vi "LABVIEW_Project.vi"() -> ()   [LabVIEW 2025]
uses:
  <vilib>/userDefined/High Color/IMAQdx.ctl
  <vilib>/MakerHub/LINX/Public/Peripherals/Analog/Analog Read 1 Chan.vi
  <vilib>/MakerHub/LINX/Public/Peripherals/Digital/Digital Write 1 Chan.vi
  <vilib>/MakerHub/LINX/Public/Peripherals/Analog/Analog Read N Chans.vi
  <vilib>/MakerHub/LINX/Public/Peripherals/Digital/Digital Write N Chans.vi
  <vilib>/MakerHub/LINX/Private/Local IO/LinxAnalogRead.vi
  <vilib>/MakerHub/LINX/Public/Utilities/Check Channel.vi
  <vilib>/MakerHub/LINX/Private/Local IO/LinxDigitalWrite.vi
  <vilib>/MakerHub/LINX/Public/Utilities/Open Serial.vi
  <vilib>/MakerHub/LINX/Private/Utilties/Generate Error.vi
  <vilib>/MakerHub/LINX/LMH-LINX.lvlib
  <vilib>/vision/driver/NI_Vision_Acquisition_Software.lvlib
panel:
  out "text":string
  in  "y":dbl=2.0 format="%#_13g"
  in  "string":string
  out "Image 2":T1(plugin-control)
  out "error out":errorcluster
  in  "Session In":T2
  out "Voltage":dbl
  out "x >= y?":bool
  in  "Serial Port":refnum<visa-resource-name>="N/A"
  in  "stop":bool
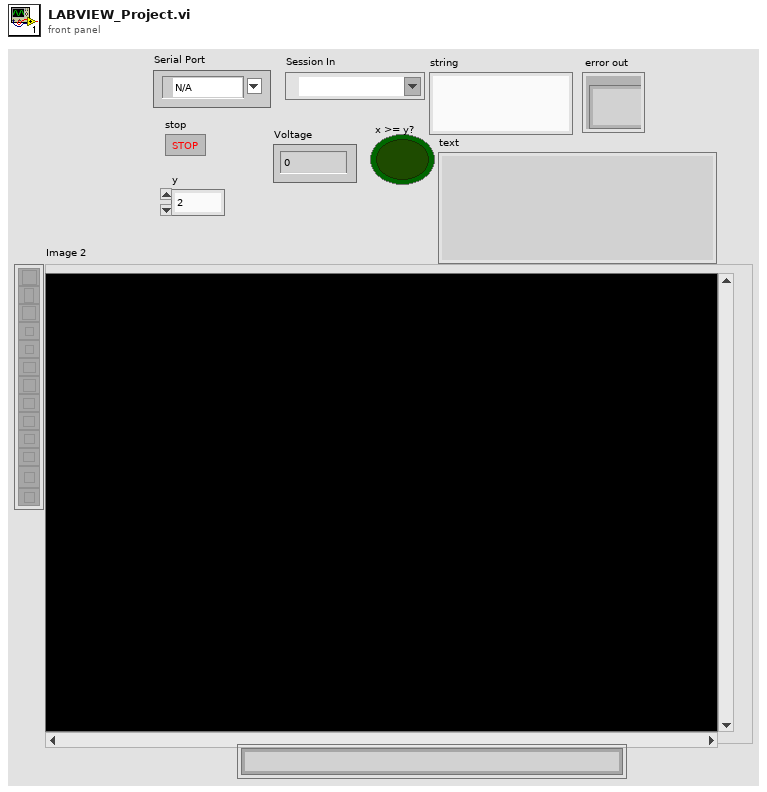
[diagram p1: front panel]
types:
  T1 = typedef "IMAQ Image.ctl" = refnum<image>
  T2 = typedef "IMAQdx.ctl" = refnum<k21>
  T3 = typedef "LMH-LINX.lvlib/LINX Ref.ctl" = cluster{"IO":T4, "Interface":T5, "LINX Device Config":T6}
  T4 = typedef "LMH-LINX.lvlib/Platform.ctl" = enum16{"Remote", "Local"}
  T5 = typedef "LMH-LINX.lvlib/Interface.ctl" = enum16{"Serial", "TCP"}
  T6 = typedef "LMH-LINX.lvlib/Device.lvlib/LINX Device Config.ctl" = cluster{"Interface":T5, "COM Port":refnum<visa-resource-name>, "TCP Configuration":T7, "Device Family":u8, "Device ID":u8, "Device Name":string, "TCP Ref":refnum<k5>, "Channels":T8}
  T7 = typedef "LMH-LINX.lvlib/Device.lvlib/TCP Config.ctl" = cluster{"IP Address":string, "Port":u16}
  T8 = typedef "LMH-LINX.lvlib/Channels.ctl" = cluster{"DI":u8[], "DO":u8[], "AI":u8[], "AO":u8[], "PWM":u8[], "QE":u8[], "UART":u8[], "I2C 2":u8[], "SPI":u8[], "CAN":u8[], "Servo":u8[], "AI Ref (V)":dbl, "AI Resolution (Bits)":u8, "AO Ref (V)":dbl, "AO Resolution (Bits)":u8}
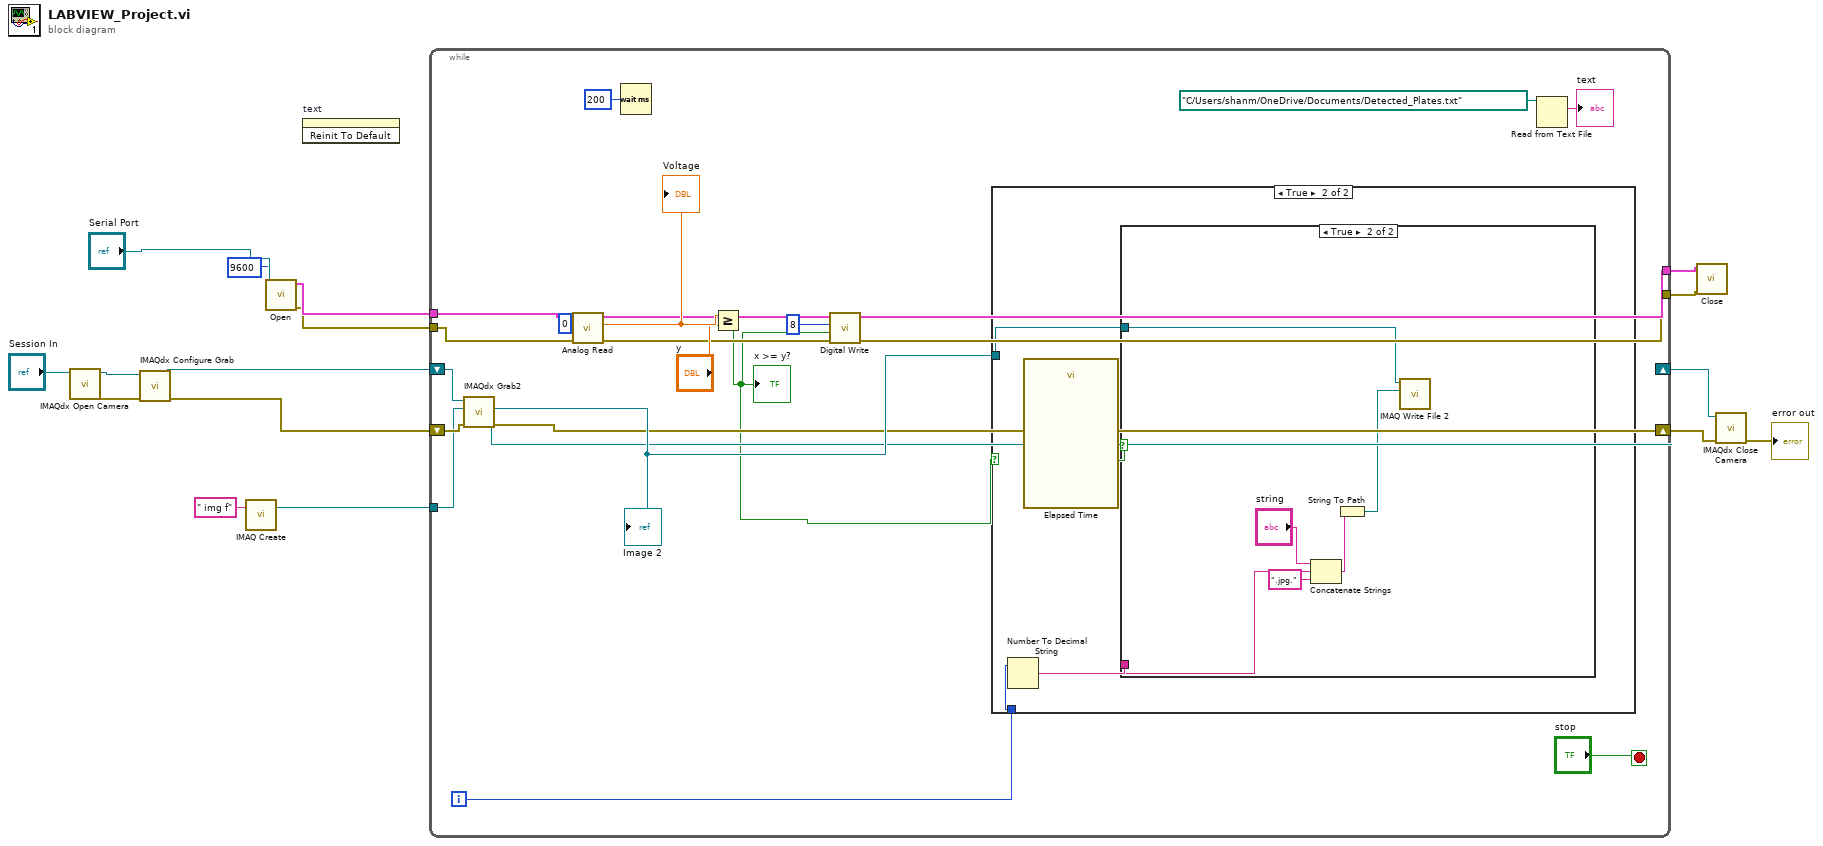
[diagram p0: block diagram]
diagram:
  n1 = call <vilib>:"IMAQdx Open Camera.vi"("Session In"="Session In") -> ("error out"=w9:errorcluster, "Session Out"=w8:T2)  [unwired: 9 in]
  n2 = call <vilib>:"IMAQdx Configure Grab.vi"("error in"=w9, "Session In"=w8) -> ("error out"=w7:errorcluster, "Session Out"=w6:T2)  [unwired: 8 in]
  n3 = call "IMAQ Create"("Image Name"=" img f") -> ("New Image"=w3:T1)  [unwired: 4 in, 1 out]
  n4 = call-poly <vilib>:"Open.vi"("Baud Rate Override"=u32 9600, "Serial Port"="Serial Port") -> ("Error Out"=w13:errorcluster, "LINX Resource"=w15:T3)  [unwired: 7 in, 1 out]
  n5 = invoke on="text" class="Str" method="Reinit To Default"() -> ()  [unwired: 3 in, 3 out]
  n6 = while {
    tunnel: w15 -> [w38]
    tunnel: [w23] -> w14
    tunnel: w13 -> [w35]
    tunnel: [w21] -> w12
    tunnel: w3 -> [w27]
    shift-right: [w26] -> w2
    shift-left: w6 -> [w29]
    shift-right: [w25] -> w1
    shift-left: w7 -> [w30]
    i -> [w28]
    stop <- "stop" stop-if-true
    n7 = call <vilib>:"IMAQdx Grab2.vi"("error in"=w30, "Image In"=w27, "Session In"=w29) -> ("error out"=w25:errorcluster, "Image Out"=w31:T1, "Session Out"=w26:T2)  [unwired: 5 in, 1 out]
    "Image 2" <- w31
    n8 = call-poly <vilib>:"Analog Read.vi"("Error In"=w35, "Analog Channel"=u8 0, "LINX Resource"=w38) -> ("Error Out"=w22:errorcluster, "Voltage"=w37:dbl, "LINX Resource"=w24:T3)  [unwired: 5 in, 1 out]
    "Voltage" <- w37
    n9 = Wait (ms)(milliseconds to wait=u32 200) -> ()  [unwired: 1 out]
    n10 = Greater Or Equal?(x=w37, y="y") -> (x >= y?=w19:bool)
    "x >= y?" <- w19
    n11 = call-poly <vilib>:"Digital Write.vi"("Error In"=w22, "Output Value"=w19, "DO Channel"=u8 8, "LINX Resource"=w24) -> ("Error Out"=w21:errorcluster, "LINX Resource"=w23:T3)  [unwired: 6 in]
    n12 = case shown="True" w19 {
      tunnel: w31 -> [_ w41]
      tunnel: w28 -> [_ w39]
      frame False {
      }
      frame True {
        n13 = Number To Decimal String(number=w39) -> (decimal integer string=w42:string)  [unwired: 1 in]
        n14 = call "Elapsed Time"() -> ("Time has Elapsed"=w40:bool)  [unwired: 12 in, 7 out]
        n15 = case shown="True" w40 {
          tunnel: w42 -> [_ w48]
          tunnel: w41 -> [_ w43]
          frame False {
          }
          frame True {
            n16 = Concatenate Strings("string", w48, ".jpg." ("string")) -> (w45:string)
            n17 = String To Path(string=w45) -> (path=w44:path)
            n18 = call-poly "IMAQ Write File 2"("File Path"=w44, "Image"=w43) -> ()  [unwired: 8 in, 2 out]
          }
        }
      }
    }
    n19 = Read from Text File(file (use dialog)=path "C:/Users/shanm/OneDrive/Documents/Detected_Plates.txt") -> (text=→"text":string)  [unwired: 3 in, 3 out]
  }
  n20 = call <vilib>:"Close.vi"("Error In"=w12, "LINX Resource"=w14) -> ()  [unwired: 9 in, 1 out]
  n21 = call <vilib>:"IMAQdx Close Camera.vi"("error in"=w1, "Session In"=w2) -> ("error out"=→"error out":errorcluster)  [unwired: 9 in]
